vi "New Timed Average Subscription.vi"(9 "Average Period [s]":dbl=1.0, 10 "Ignore Past Updates? (F)":bool, 11 "TimedAverageSubscription In":refnum<class "TimedAverageSubscription.lvclass">) -> (3 "TimedAverageSubscription Out":refnum<class "TimedAverageSubscription.lvclass">)   [LabVIEW 2015, in "SubscriptionPolicy.lvlib" / "TimedAverageSubscription.lvclass"]
uses:
  TimedAverageSubscription.lvclass
  TimedAverageSubscription.lvclass/TimedAverageSubscription.ctl
  Components/TimedAverageBuffer/TimedAverageBuffer.lvclass
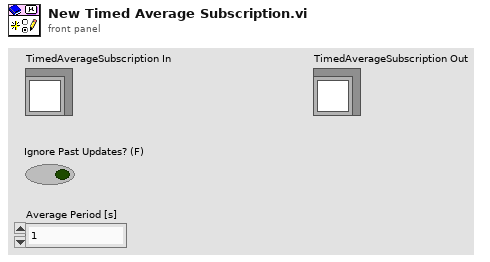
[diagram p1: front panel]
types:
  T1 = typedef "TimedAverageBuffer.lvlib/TimedAverageBuffer.lvclass/TimedAverageBuffer Reference.ctl" = refnum<data-value>
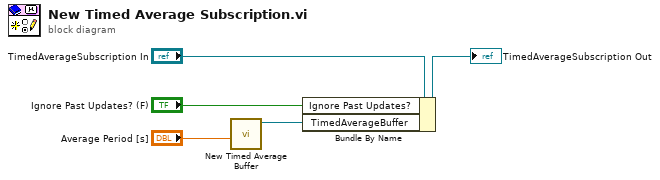
[diagram p0: block diagram]
diagram:
  n1 = call "New Timed Average Buffer.vi"("Buffer Duration [s]"="Average Period [s]") -> ("Timed Average Buffer"=w1:T1)  [unwired: 9 in, 1 out]
  n2 = Bundle By Name(cluster="TimedAverageSubscription In", "Ignore Past Updates?"="Ignore Past Updates? (F)", "TimedAverageBuffer"=w1) -> (→"TimedAverageSubscription Out":refnum<class "TimedAverageSubscription.lvclass">)
